vi "Vector Field Controler.vi"(7 "Initialize?":bool, 8 "obstacle clearance (m)":dbl) -> (0 "VTan_Cmd":dbl(slide) scale=-10.0..10.0, 3 "Command Heading":dbl)   [LabVIEW 2012]
panel:
  out "histogram out":dbl[](array[numeric])
  in  "outer threshold":dbl=1.1
  in  "inner threshold":dbl=0.6
  in  "max speed":dbl=0.4
  out "Bearing":dbl
  out "Target Distance":dbl
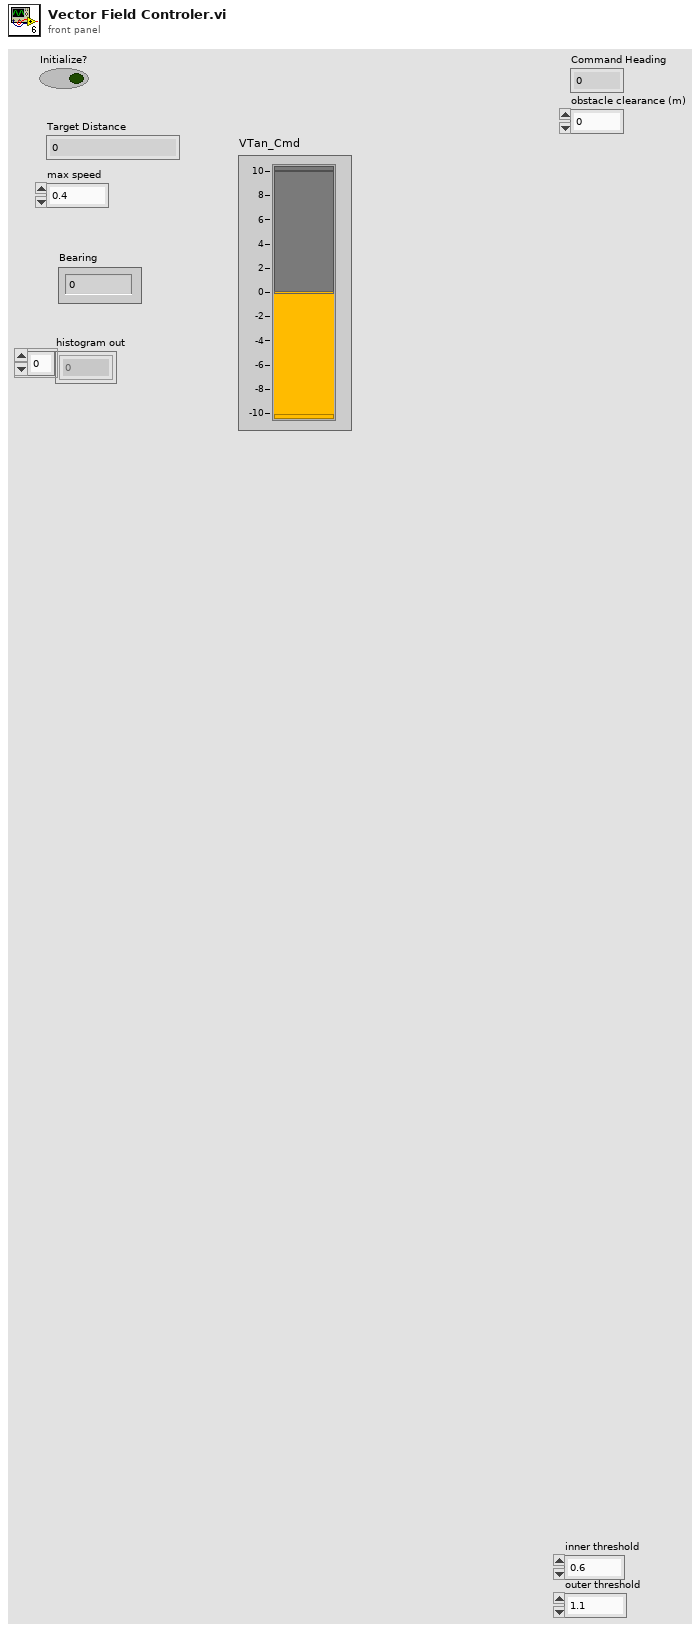
[diagram p1: front panel]
types:
  T1 = cluster{"Position":cluster{"Roll":dbl, "Pitch":dbl, "Yaw":dbl}, "Orientation Matrix":dbl[][], "Magnetic Field":cluster{"Z-Axis Magnetic Field":dbl, "Y-Axis Magnetic Field":dbl, "X-Axis Magnetic Field":dbl}, "Acceleration":cluster{"Z-Axis Acceleration":dbl, "Y-Axis Acceleration":dbl, "X-Axis Acceleration":dbl}, "Angular Rate":cluster{"X-Axis Angular Rate":dbl, "Y-Axis Angular Rate":dbl, "Z-Axis Angular Rate":dbl}, "Quaternion":dbl[]}
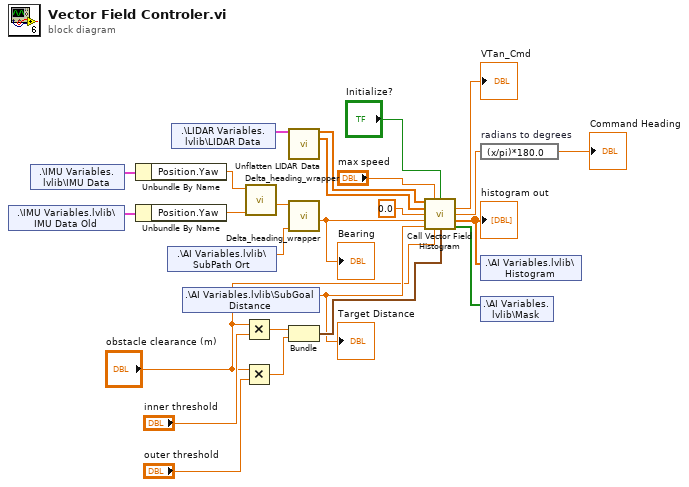
[diagram p0: block diagram]
diagram:
  n1 = shared-variable ".\\IMU Variables.lvlib\\IMU Data Old"() -> (w9:T1)  [unwired: 1 in, 1 out]
  n2 = shared-variable ".\\IMU Variables.lvlib\\IMU Data"() -> (w25:T1)  [unwired: 1 in, 1 out]
  n3 = Unbundle By Name(w25) -> ("Position.Yaw"=w24:dbl)
  n4 = Unbundle By Name(w9) -> ("Position.Yaw"=w8:dbl)
  n5 = shared-variable ".\\AI Variables.lvlib\\SubPath Ort"() -> (w6:dbl)  [unwired: 1 in, 1 out]
  n6 = shared-variable ".\\LIDAR Variables.lvlib\\LIDAR Data"() -> (w22:cluster{"Magnitude":dbl[], "Direction":dbl[]})  [unwired: 1 in, 1 out]
  n7 = shared-variable ".\\AI Variables.lvlib\\SubGoal Distance"() -> (w10:dbl)  [unwired: 1 in, 1 out]
  "Target Distance" <- w10
  n8 = Multiply(x="obstacle clearance (m)", y="inner threshold") -> (x*y=w17:dbl)
  n9 = Multiply(x="obstacle clearance (m)", y="outer threshold") -> (x*y=w16:dbl)
  n10 = call "Delta_heading_wrapper.vi"("Goal Heading"=w8, "Robot Heading"=w24) -> ("Heading Adjustment"=w7:dbl)  [unwired: 9 in]
  n11 = call "Unflatten LIDAR Data.vi"("LIDAR Data"=w22) -> ("Range (m)"=w21:dbl[], "Bearing (rad)"=w20:dbl[])  [unwired: 13 in]
  n12 = call "Delta_heading_wrapper.vi"("Goal Heading"=w6, "Robot Heading"=w7) -> ("Heading Adjustment"=w5:dbl)  [unwired: 9 in]
  "Bearing" <- w5
  n13 = Bundle(w17, w16) -> (w15:cluster{dbl, dbl})  [unwired: 1 in]
  n14 = call "Call Vector Field Histogram.vi"("LIDAR magn. (m)"=w21, "max speed"="max speed", "Initialize?"="Initialize?", "LIDAR angle (rad)"=w20, "current heading (rad)"=0.0, "target heading (rad)"=w5, "target distance"=w10, "obstacle clearance (m)"="obstacle clearance (m)", "thresholds"=w15) -> ("command vy"=→"VTan_Cmd":dbl, "command heading (rad)"=w4:dbl, "histogram out"=w12:dbl[], "mask out"=w14:bool[])  [unwired: 2 in, 1 out]
  "histogram out" <- w12
  n15 = expression code="(x/pi)*180.0" "radians to degrees"(w4) -> (→"Command Heading":dbl)
  n16 = shared-variable ".\\AI Variables.lvlib\\Histogram"(w12) -> ()  [unwired: 1 in, 1 out]
  n17 = shared-variable ".\\AI Variables.lvlib\\Mask"(w14) -> ()  [unwired: 1 in, 1 out]
